vi "LM_fit.vi"(4 "Salinity":dbl, 5 "HCl Concentration":dbl, 6 "k":dbl, 7 "Corrected Cell Temperature Mean":dbl, 8 "m/m0":dbl[](array[numeric]), 9 "TA estimate":dbl, 10 "H+ estimate":dbl[](array[numeric]), 11 "E0 estimate":dbl format="%.2f") -> (0 "mse":dbl format="%.4e", 1 "FitE0":dbl, 3 "FitAlk":dbl)   [LabVIEW 2010]
uses:
  <vilib>/gmath/NumericalOptimization/Nonlinear Curve Fit LM formula string.vi
  <vilib>/gmath/NI_Gmath.lvlib
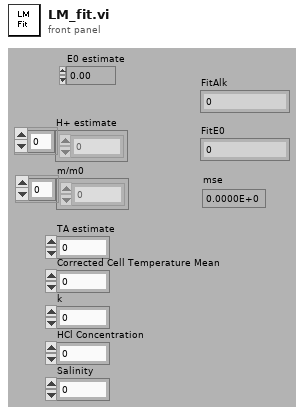
[diagram p1: front panel]
types:
  T1 = cluster{"model":string, "Parameters":string[], "x":string}
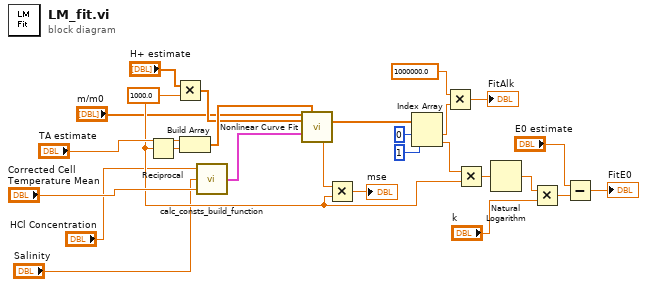
[diagram p0: block diagram]
diagram:
  w12 = 1000.0 ("y")
  n1 = Reciprocal(x=w12) -> (1/x=w21:dbl)
  n2 = Multiply(x="H+ estimate", y=w12) -> (x*y=w9:dbl[])
  n3 = Build Array("TA estimate", w21) -> (w10:dbl[])
  n4 = call "calc_consts_build_function.vi"("Corrected Cell Temperature Mean"="Corrected Cell Temperature Mean", "Salinity"="Salinity", "HCl Concentration"="HCl Concentration") -> ("model description"=w11:T1)
  n5 = call-poly <vilib>:"Nonlinear Curve Fit.vi"("Y"="m/m0", "initial parameters"=w10, "X"=w9, "model description"=w11) -> ("best fit parameters"=w6:dbl[], "residue"=w7:dbl)  [unwired: 7 in, 3 out]
  n6 = Multiply(x=w7, y=w12) -> (x*y=→"mse":dbl)
  n7 = Index Array(array=w6, index #1=0 ("Index"), index #2=1 ("Index")) -> (element #1=w25:dbl, element #2=w4:dbl)
  n8 = Multiply(x=1000000.0 ("y"), y=w25) -> (x*y=→"FitAlk":dbl)
  n9 = Multiply(x=w4, y=w12) -> (x*y=w18:dbl)
  n10 = Natural Logarithm(1:w18) -> (0:w20:dbl)
  n11 = Multiply(x=w20, y="k") -> (x*y=w19:dbl)
  n12 = Subtract(x="E0 estimate", y=w19) -> (x-y=→"FitE0":dbl)
